vi "PH_PILS.PC _Boolean.vi"(0 "i ref in":refnum<vi>, 2 "serviceName":string, 3 "Value":i32, 5 "error IO":errorcluster) -> (14 "i ref out":refnum<vi>, 19 "error out":errorcluster)   [LabVIEW 2014, in "PH_PILS.lvlib"]
doc: "This is the proc case \"_Boolean\"."
uses:
  PH_PILS.lvlib
  PH_Basics/PH_Common/PH_Common.lvlib
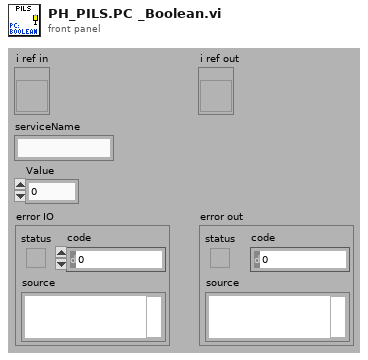
[diagram p1: front panel]
types:
  T1 = typedef "PH_PILS.lvlib/PH_PILS.i attribute.ctl" = cluster{"Boolean":cluster{"GUI Ref":refnum<vi>, "Status":i32}[], "GUI Refs Exp. Shutters":cluster{"1":refnum<vi>, "2":refnum<vi>, "3":refnum<vi>, "4":refnum<vi>}, "Tristate2Run GUI Refs":refnum<vi>[], "EO-Likes":cluster{"GUI Ref":refnum<vi>, "Status":i32}[], "Operation Mode":cluster{"Operation Mode":T2, "GUI":cluster{"Ref State":refnum<vi>, "Ref":refnum<vi>}, "Servicemode":cluster{"Tagname":string, "Status":i32}, "Labormode":cluster{"Tagname":string, "Status":i32}, "Searchmode":cluster{"Tagname":string, "Status":i32}, "Shotmode":cluster{"Tagname":string, "Status":i32}}, "Submode":cluster{"Submode":T3, "GUI":cluster{"Ref State":refnum<vi>, "Ref":refnum<vi>}, "Submode":cluster{"Tagname":string, "Status":i32}}, "Experiment":cluster{"Experiment":enum16{"unknown", "intern", "4 (Z6)", "3", "2", "1"}, "GUI":cluster{"Ref State":refnum<vi>, "Ref":refnum<vi>}, "intern":cluster{"Tagname":string, "Status":i32}, "Exp 4":cluster{"Tagname":string, "Status":i32}, "Exp 3":cluster{"Tagname":string, "Status":i32}, "Exp 2":cluster{"Tagname":string, "Status":i32}, "Exp 1":cluster{"Tagname":string, "Status":i32}}, "TristateNormal":cluster{"GUI Ref":refnum<vi>, "Status":i32}[], "Door Tags":cluster{"GUI Ref":refnum<vi>, "Status":i32}[], "GUIlessTags":cluster{"Name":string, "Status":i32}[], "Beamline GUI Refs":refnum<vi>[], "Special Boolean":cluster{"GUI Ref":refnum<vi>, "Status":i32}[], "Laserpower":cluster{"GUI Ref":refnum<vi>, "Status":i32}[], "Shutter":cluster{"GUI Ref":refnum<vi>, "Status":i32}[], "Tristate EO Like":cluster{"GUI Ref":refnum<vi>, "Status":i32}[], "PP":cluster{"GUI Ref":refnum<vi>, "Status":i32, "Head Ref":refnum<vi>, "Slider Ref":refnum<vi>}[], "Switch Knobs":cluster{"GUI Ref":refnum<vi>, "Status":i32}[], "Latch Knob GUI Refs":refnum<vi>[], "FailureCounter":i32, "Enabled Status":cluster{"Laser":i32, "PreAmp":i32, "MainAmp":i32}, "Mercury":refnum<vi>, "Instance Rods":string, "Logfile":path, "Beckhoff-Instance Internal":string, "Beckhoff-Instance External":string, "Enabling Rights":cluster{"Name":string, "Password":string, "PA?":bool, "MA?":bool, "Exp?":bool}[]}
  T2 = typedef "PH_PILS.lvlib/PH_PILS.Operation Mode.ctl" = enum16{"unknown", "Service", "Labor", "Search", "Shot"}
  T3 = typedef "PH_PILS.lvlib/PH_PILS.Submode.ctl" = enum16{"unknown", "HV-Normal", "HV-Test"}
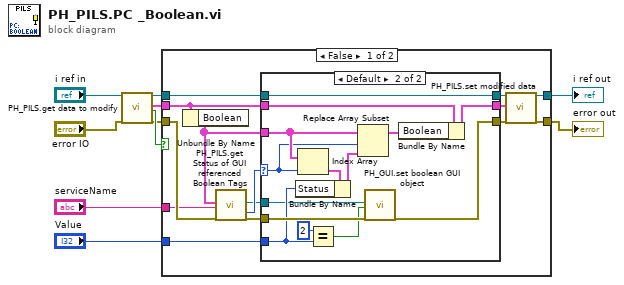
[diagram p0: block diagram]
diagram:
  n1 = call "PH_PILS.get data to modify.vi"("i ref in"="i ref in", "error in (no error)"="error IO") -> ("i ref out"=w5:refnum<vi>, "i attribute"=w8:T1, "timed out"=w10:bool, "error out"=w6:errorcluster)  [unwired: 14 in]
  n2 = case shown="False" w10 {
    tunnel: w5 -> [w24 w43]
    tunnel: [w18 w43] -> w2
    tunnel: [w21 w42] -> w1
    tunnel: w6 -> [w15 w42]
    tunnel: "serviceName" -> [w14 _]
    tunnel: w8 -> [w23 _]
    tunnel: "Value" -> [w22 _]
    frame False {
      n3 = Unbundle By Name(w23) -> ("Boolean"=w16:cluster{"GUI Ref":refnum<vi>, "Status":i32}[])
      n4 = call "PH_PILS.get Status of GUI referenced Boolean Tags.vi"("Tags"=w16, "Tagname"=w14, "error in"=w15) -> ("GUI Ref"=w11:refnum<vi>, "index of element"=w13:i32, "error out"=w12:errorcluster)  [unwired: 13 in, 1 out]
      n5 = case shown="Default" w13 {
        selector: w13 -> [_ w32]
        tunnel: w24 -> [w27 w31]
        tunnel: [w27 w31] -> w19
        tunnel: [w26 w29] -> w20
        tunnel: w12 -> [w26 w39]
        tunnel: w16 -> [_ w40]
        tunnel: w23 -> [w25 w38]
        tunnel: w22 -> [_ w34]
        tunnel: [w25 w30] -> w17
        tunnel: w11 -> [_ w28]
        frame -1 {
        }
        frame Default {
          n6 = Index Array(array=w40, index=w32) -> (element=w33:cluster{"GUI Ref":refnum<vi>, "Status":i32})
          n7 = Bundle By Name(cluster=w33, "Status"=w34) -> (w35:cluster{"GUI Ref":refnum<vi>, "Status":i32})
          n8 = Equal?(x=2 ("y"), y=w34) -> (x = y?=w37:bool)
          n9 = Replace Array Subset(array=w40, new element=w35, index=w32) -> (w41:cluster{"GUI Ref":refnum<vi>, "Status":i32}[])
          n10 = call "PH_GUI.set boolean GUI object.vi"("Boolean Knob GUI Ref"=w28, "Value"=w37, "error in (no error)"=w39) -> ("error out"=w29:errorcluster)  [unwired: 16 in]
          n11 = Bundle By Name(cluster=w38, "Boolean"=w41) -> (w30:T1)
        }
      }
      n12 = call "PH_PILS.set modified data.vi"("i ref in"=w19, "i attribute"=w17, "error in (no error)"=w20) -> ("i ref out"=w18:refnum<vi>, "error out"=w21:errorcluster)  [unwired: 15 in]
    }
    frame True {
    }
  }
  "error out" <- w1
  "i ref out" <- w2
